vi "Init.vi"(11 "error in (no error)":errorcluster) -> (4 "Nikon cluster":T1, 6 "C-867-cluster":T3, 8 "E-709-cluster":T2, 15 "error out":errorcluster)   [LabVIEW 2014]
doc: "This VI initializes the Nikon TI2 microscope, the PI C-867 XY stage and the PI E-709 Z stage"
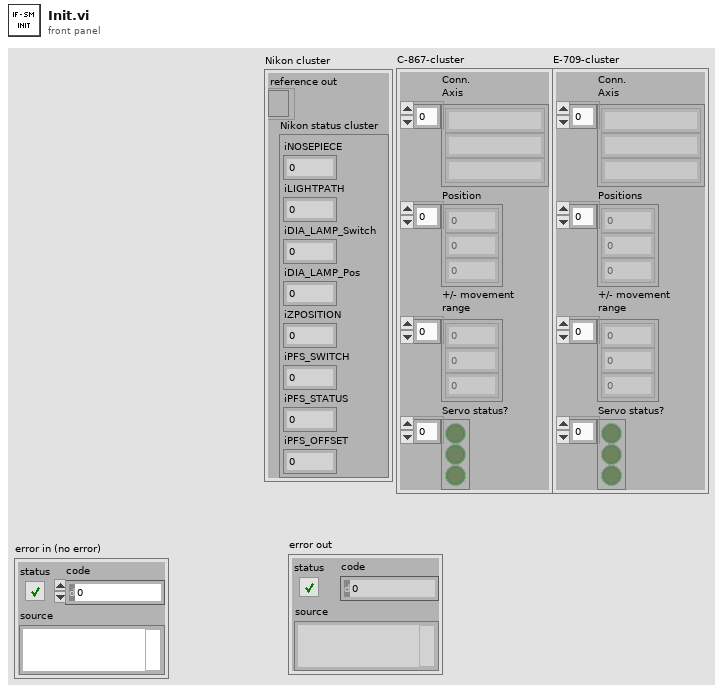
[diagram p1: front panel]
types:
  T1 = cluster{"reference out":refnum<k7>, "Nikon status cluster":cluster{"iNOSEPIECE":i32, "iLIGHTPATH":i32, "iDIA_LAMP_Switch":i32, "iDIA_LAMP_Pos":i32, "iZPOSITION":i32, "iPFS_SWITCH":i32, "iPFS_STATUS":i32, "iPFS_OFFSET":i32}}
  T2 = cluster{"Conn. \nAxis":string[], "Positions":dbl[], "+/- movement\nrange":dbl[], "Servo status?":bool[]}
  T3 = cluster{"Conn. \nAxis":string[], "Position":dbl[], "+/- movement\nrange":dbl[], "Servo status?":bool[]}
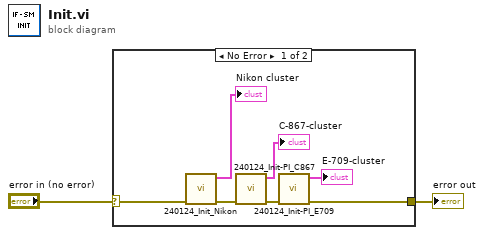
[diagram p0: block diagram]
diagram:
  n1 = case shown="No Error" "error in (no error)" {
    selector: "error in (no error)" -> [w3 w10]
    tunnel: [w4 w10] -> w1
    frame No Error {
      n2 = call "240124_Init_Nikon.vi"("error in (no error)"=w3) -> ("error out"=w8:errorcluster, "Nikon cluster"=→"Nikon cluster":T1)  [unwired: 9 in]
      n3 = call "240124_Init-PI_C867.vi"("error in (no error)"=w8) -> ("error out"=w9:errorcluster, "C-867-cluster"=→"C-867-cluster":T3)  [unwired: 9 in]
      n4 = call "240124_Init-PI_E709.vi"("error in (no error)"=w9) -> ("error out"=w4:errorcluster, "E-709-cluster"=→"E-709-cluster":T3)  [unwired: 9 in]
    }
    frame Error {
    }
  }
  "error out" <- w1
